vi "setROI.vi"(8 "error in (no error)":errorcluster, 11 "FTTclusterIn":T1) -> (0 "error out":errorcluster, 3 "FTTclusterOut":T1)   [LabVIEW 2016]
uses:
  controls/UI Data.ctl
  Program Files (x86)/National Instruments/LabVIEW 2015/user.lib/cameraLibrary/cameraLibrary.lvlib
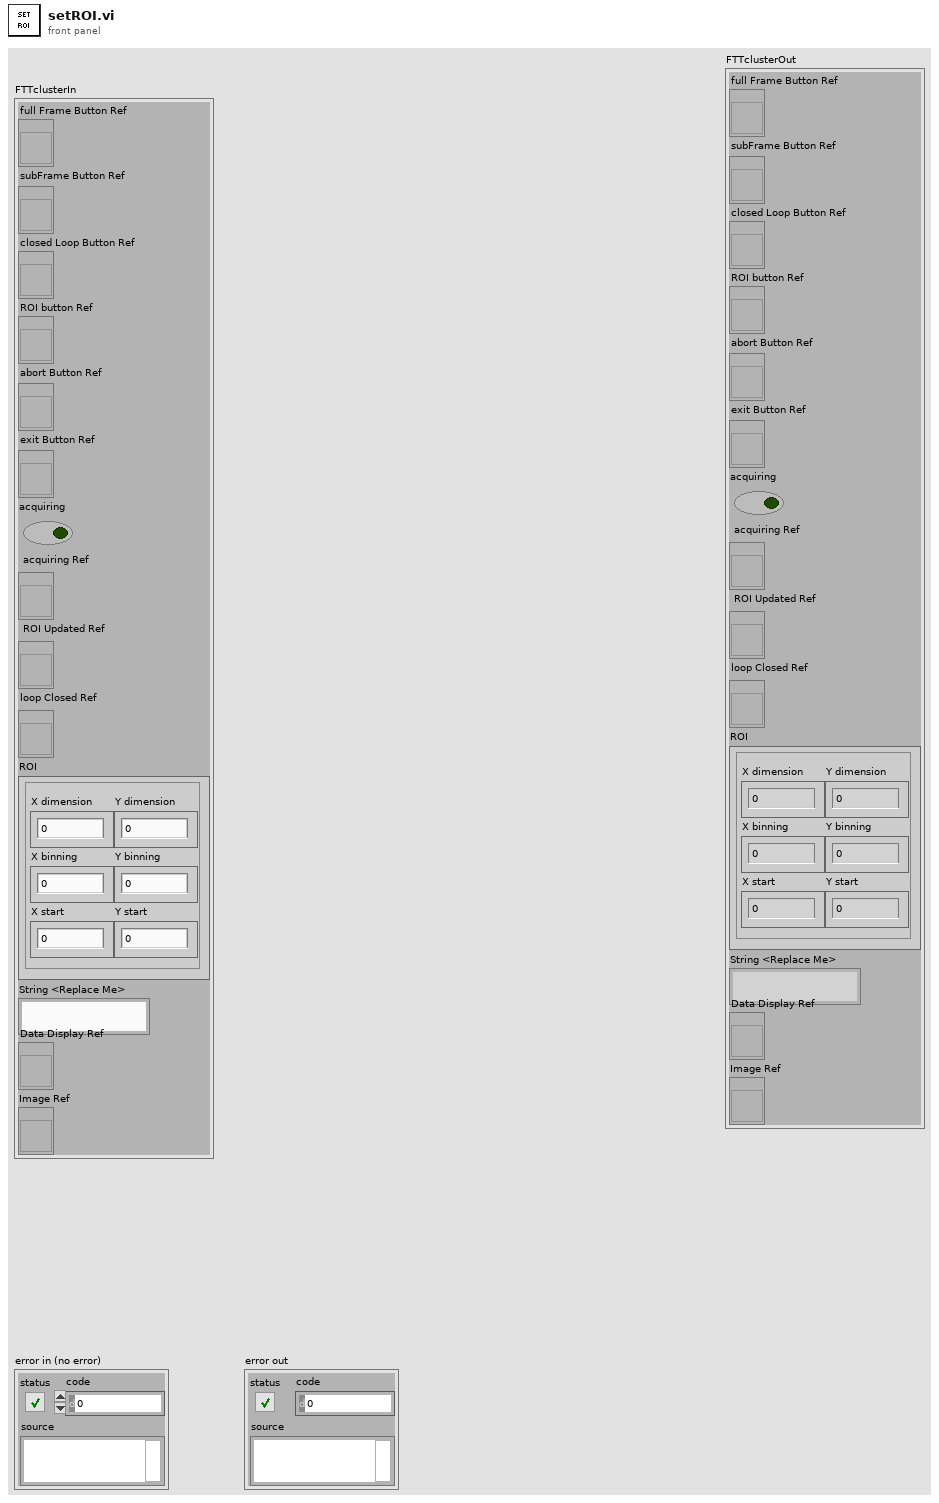
[diagram p1: front panel]
types:
  T1 = typedef "UI Data.ctl" = cluster{"full Frame Button Ref":refnum<vi>, "subFrame Button Ref":refnum<vi>, "closed Loop Button Ref":refnum<vi>, "ROI button Ref":refnum<vi>, "abort Button Ref":refnum<vi>, "exit Button Ref":refnum<vi>, "acquiring":bool, " acquiring Ref":refnum<vi>, " ROI Updated Ref":refnum<vi>, "loop Closed Ref":refnum<vi>, "ROI":cluster{"X dimension":i16, "Y dimension":i16, "X binning":i16, "Y binning":i16, "X start":i16, "Y start":i16}, "String <Replace Me>":string, "Data Display Ref":refnum<vi>, "Image Ref":refnum<vi>}
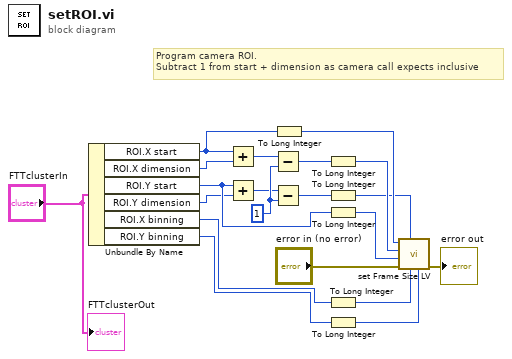
[diagram p0: block diagram]
diagram:
  w12 = i16 1 ("y")
  # "Program camera ROI.\nSubtract 1 from start + dimension as camera call expects inclusive"
  n1 = Unbundle By Name("FTTclusterIn") -> ("ROI.X start"=w15:i16, "ROI.X dimension"=w2:i16, "ROI.Y start"=w17:i16, "ROI.Y dimension"=w3:i16, "ROI.X binning"=w6:i16, "ROI.Y binning"=w8:i16)
  n2 = Add(x=w15, y=w2) -> (x+y=w10:i16)
  n3 = Add(x=w17, y=w3) -> (x+y=w11:i16)
  n4 = Subtract(x=w10, y=w12) -> (x-y=w20:i16)
  n5 = Subtract(x=w11, y=w12) -> (x-y=w13:i16)
  n6 = To Long Integer(number=w15) -> (32bit integer=w16:i32)
  n7 = To Long Integer(number=w20) -> (32bit integer=w19:i32)
  n8 = To Long Integer(number=w13) -> (32bit integer=w14:i32)
  n9 = To Long Integer(number=w17) -> (32bit integer=w18:i32)
  n10 = To Long Integer(number=w6) -> (32bit integer=w7:i32)
  n11 = To Long Integer(number=w8) -> (32bit integer=w9:i32)
  n12 = call "set Frame Size LV.vi"("vbin"=w9, "hbin"=w7, "vend"=w14, "error in (no error)"="error in (no error)", "vstart"=w18, "hend"=w19, "hstart"=w16) -> ("error out"=→"error out":errorcluster)  [unwired: 4 in]
  "FTTclusterOut" <- "FTTclusterIn"
